vi "Parse Recipe.vi"(10 "Get Recipe reply JSON":string) -> (1 "Array":T1[](array[typedef]), 2 "Recipe":string[](array[string]))   [LabVIEW 2021]
uses:
  PPLs/Recipe.lvlibp/Controls/Fixed Parameters.ctl
  dae2f689-941e-4efe-8cf1-ce7ba08b26b2.vi
  bd70a2ca-1625-48ae-a1ff-43d5301d01ec.vi
  0e9874e1-ca7b-49d1-bf08-ee78fea6aba5.vi
  5fdde2c3-a312-4f36-9cde-9d716aa16c2f.vi
  a0b9bacf-30f6-44f9-83db-e56ac0b0af33.vi
  <vilib>/JDP Science/JSONtext/Next JSON Value.vi
  <vilib>/JDP Science/JSONtext/String Subset.vi
  <vilib>/JDP Science/JSONtext/Parsing/Advance past next JSON Value (inlined COPY).vi
  <vilib>/JDP Science/JSONtext/Parsing/Advance past whitespace.vi
  <vilib>/JDP Science/JSONtext/Parsing/Advance past String.vi
  <vilib>/JDP Science/JSONtext/Parsing/Advance past Number.vi
  <vilib>/JDP Science/JSONtext/Parsing/Advance past Line Ending.vi
  <vilib>/JDP Science/JSONtext/Parsing/Parse Full Path or Item Name.vi
  <vilib>/JDP Science/JSONtext/Parsing/Advance past Array.vi
  <vilib>/JDP Science/JSONtext/Parsing/Advance past Object.vi
  <vilib>/JDP Science/JSONtext/support/Error Cluster From Code.vi
  <vilib>/JDP Science/JSONtext/Offset/Find Item Locations by Path.vi
  <vilib>/JDP Science/JSONtext/JSON text to Variant.vi
  <vilib>/JDP Science/JSONtext/LVClass Serializer/JSONtext LVClass Serializer.lvclass
  <vilib>/JDP Science/JSONtext/JSONtext.lvlib
  PPLs/Recipe.lvlibp/Classes/Recipe/Recipe.lvclass
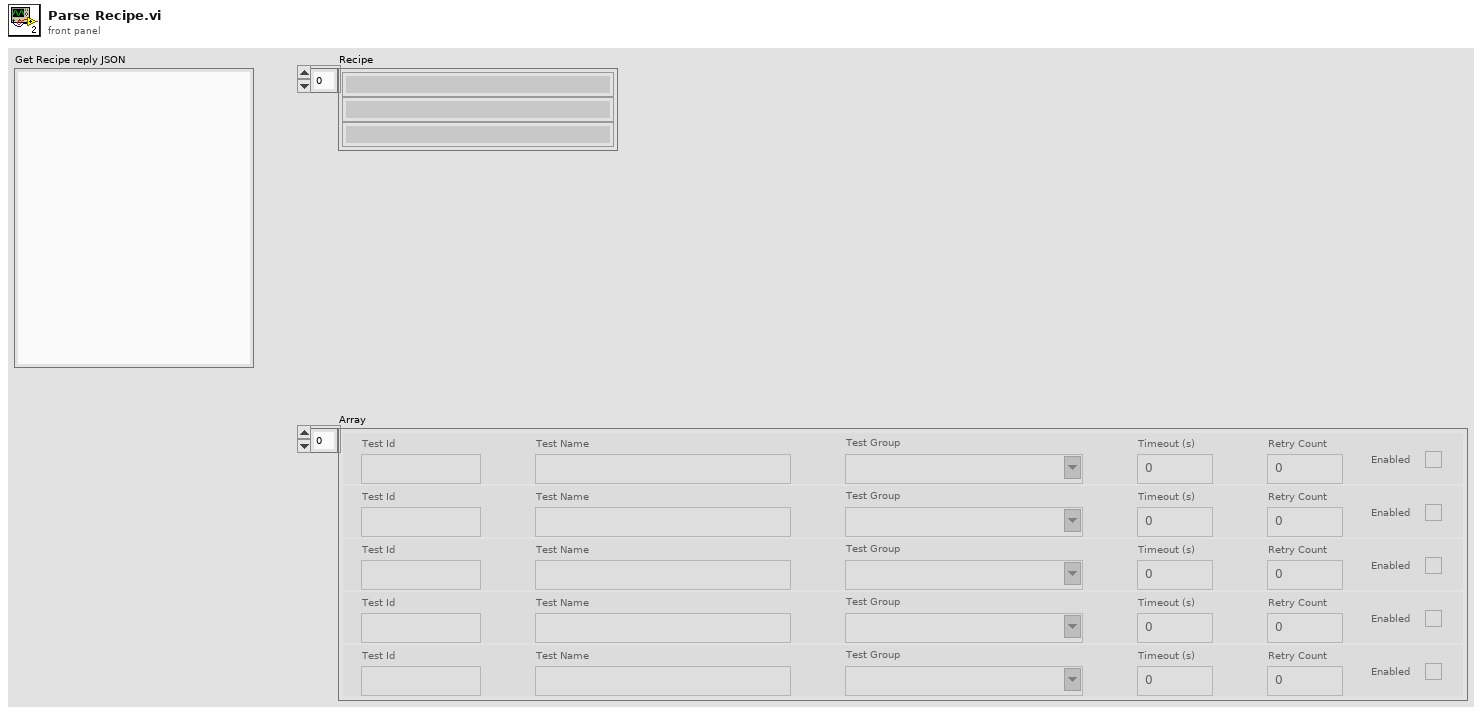
[diagram p1: front panel]
types:
  T1 = typedef "Recipe.lvlibp/Recipe.lvclass/Fixed Parameters.ctl" = cluster{"Test Id":string, "Test Name":string, "Test Group":string, "Timeout (s)":u16, "Retry Count":u16, "Enabled":bool}
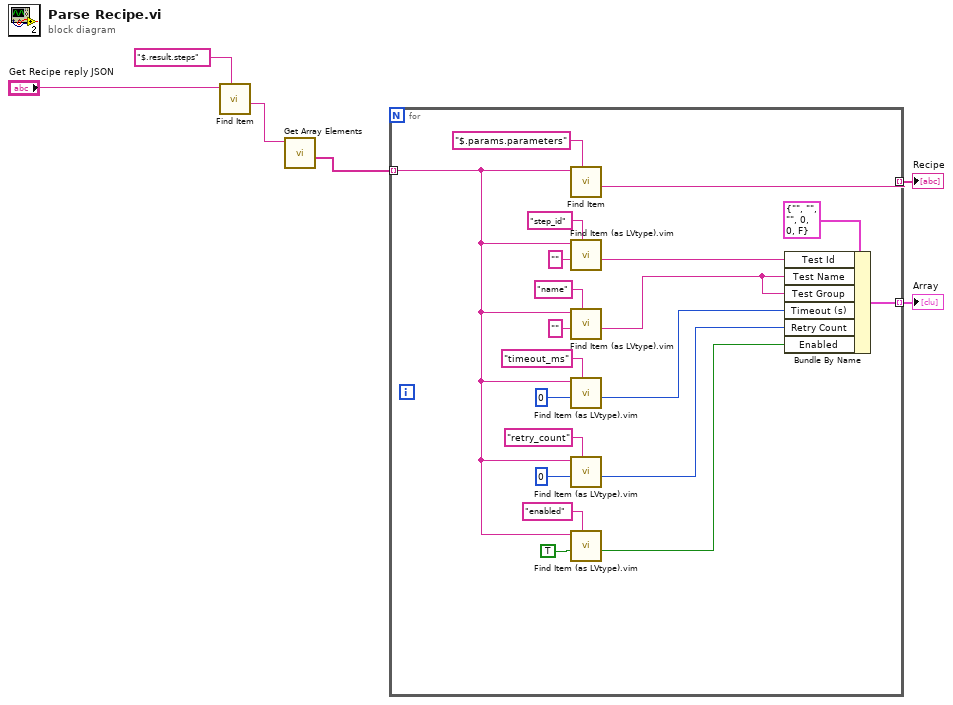
[diagram p0: block diagram]
diagram:
  n1 = call <vilib>:"Find Item.vi"("$Path or Item Name"="$.result.steps", "JSON"="Get Recipe reply JSON") -> ("<JSON>"=w4:string)  [unwired: 6 in, 3 out]
  n2 = call <vilib>:"Get Array Elements.vi"("JSON"=w4) -> ("<JSON>"=w3:string[])  [unwired: 8 in, 2 out]
  n3 = for {
    tunnel: w3 -> [w10] mode=indexing
    tunnel: [w25] -> w2 mode=indexing
    tunnel: [w7] -> w1 mode=indexing
    n4 = call <vilib>:"Find Item.vi"("$Path or Item Name"="$.params.parameters", "JSON"=w10) -> ("<JSON>"=w25:string)  [unwired: 6 in, 3 out]
    n5 = call "Find Item (as LVtype).vim"("$Path or Item Name"="step_id", "Data Type and Default Value"="", "JSON"=w10) -> ("Data"=w21:string)  [unwired: 5 in, 3 out]
    n6 = call "Find Item (as LVtype).vim"("$Path or Item Name"="name", "Data Type and Default Value"="", "JSON"=w10) -> ("Data"=w18:string)  [unwired: 5 in, 3 out]
    n7 = call "Find Item (as LVtype).vim"("$Path or Item Name"="timeout_ms", "Data Type and Default Value"=u16 0 ("Timeout (s)"), "JSON"=w10) -> ("Data"=w15:u16)  [unwired: 5 in, 3 out]
    n8 = call "Find Item (as LVtype).vim"("$Path or Item Name"="retry_count", "Data Type and Default Value"=u16 0 ("Timeout (s)"), "JSON"=w10) -> ("Data"=w12:u16)  [unwired: 5 in, 3 out]
    n9 = call "Find Item (as LVtype).vim"("$Path or Item Name"="enabled", "Data Type and Default Value"=TRUE, "JSON"=w10) -> ("Data"=w8:bool)  [unwired: 5 in, 3 out]
    n10 = Bundle By Name(cluster=T1 {"Test Id"="", "Test Name"="", "Test Group"="", "Timeout (s)"=0, "Retry Count"=0, "Enabled"=FALSE} ("Fixed Parameters"), "Test Id"=w21, "Test Name"=w18, "Test Group"=w18, "Timeout (s)"=w15, "Retry Count"=w12, "Enabled"=w8) -> (w7:T1)
  }
  "Recipe" <- w2
  "Array" <- w1
